vi "case_update_printer.vi"(0 "VISA resource name in":refnum<visa-resource-name>, 1 "Main VI reference":refnum<vi>, 5 "Refnum in":T2, 7 "message cluster":T1, 9 "initialized":bool, 11 "error in (no error)":errorcluster) -> (6 "Refnum out":T2, 8 "initialized out":bool, 15 "error out":errorcluster)   [LabVIEW 2020]
uses:
  <vilib>/Utility/config.llb/Config Data RefNum.ctl
  controls/message cluster.ctl
  64326d8d-66cc-4468-9ae1-7dc234c258b1.vi
  abe03f72-a603-4dcd-809d-10ef4235ec58.vi
  b926d721-a196-43c8-96cf-a21578f52920.vi
  db0f2e50-7a24-4501-afe9-f92d5168bb2c.vi
  168b0aa5-e037-40d0-9813-dbd61d4aeaf3.vi
  a9cd6c2e-b2c6-430f-85e8-9fbb4aaab0bd.vi
  13e36b39-ac3a-4ec8-9f6e-05db5e58b898.vi
  b8b0c841-a67c-40df-9bde-ad31628f9d82.vi
  <vilib>/Utility/config.llb/Read Key (String).vi
  <vilib>/Utility/config.llb/Read Key (Double).vi
  <vilib>/Utility/config.llb/NI_LVConfig.lvlib
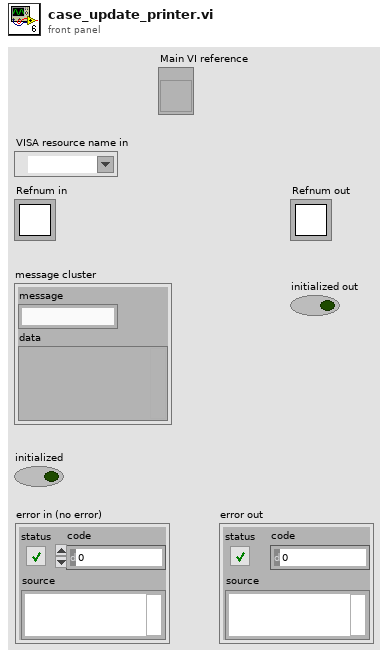
[diagram p1: front panel]
types:
  T1 = typedef "message cluster.ctl" = cluster{"message":string, "data":variant}
  T2 = typedef "NI_LVConfig.lvlib/Config Data RefNum.ctl" = refnum<k1>
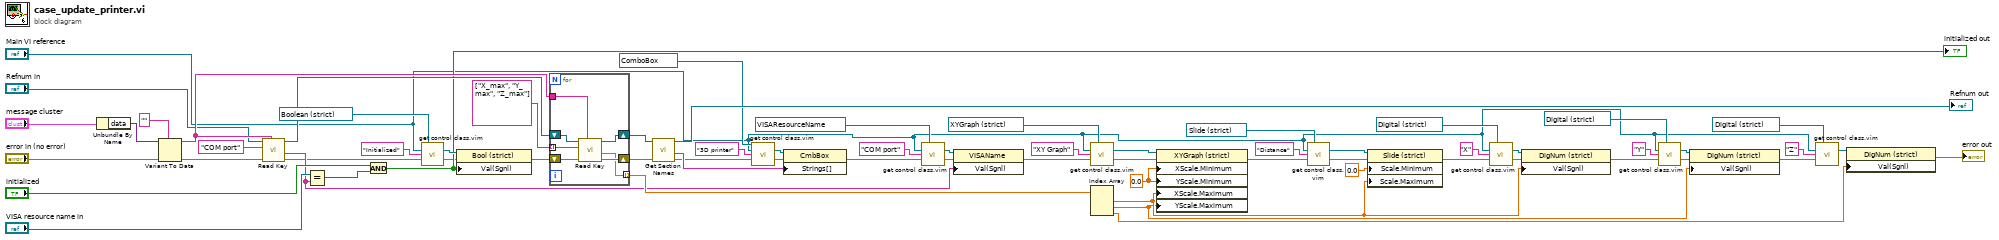
[diagram p0: block diagram]
diagram:
  w64 = 0.0 ("X Scale.Range:Minimum")
  n1 = Unbundle By Name("message cluster") -> ("data"=w47:variant)
  n2 = Variant To Data(error in="error in (no error)", type="", Variant=w47) -> (data=w57:string, error out=w50:errorcluster)
  n3 = call-poly <vilib>:"Read Key.vi"("section"=w57, "error in (no error)"=w50, "key"="COM port", "refnum"="Refnum in") -> ("error out"=w4:errorcluster, "value"=w15:string, "refnum out"=w56:T2)  [unwired: 4 in, 1 out]
  n4 = Equal?(x="VISA resource name in", y=w15) -> (x = y?=w63:bool)
  n5 = And(x="initialized", y=w63) -> (x .and. y?=w6:bool)
  "initialized out" <- w6
  n6 = call "get control class.vim"("Control class"=refnum<vi> refnum ("Initialized"), "Main VI reference"="Main VI reference", "Label"="Initialized", "error in (no error)"=w4) -> ("Control out"=w8:refnum<vi>, "error out"=w3:errorcluster)  [unwired: 10 in]
  n7 = property on="Property Node" class="Bool (strict)"(reference=w8, error in=w3, "Val(Sgnl)"=w6) -> (error out=w2:errorcluster)  [unwired: 1 out]
  n8 = for {
    tunnel: string[] ["X_max", "Y_max", "Z_max"] -> [w74] mode=indexing
    shift-right: [w71] -> w61
    shift-left: w2 -> [w72]
    shift-right: [w70] -> w59
    shift-left: w56 -> [w73]
    tunnel: [w69] -> w53 mode=indexing
    tunnel: w57 -> [w68]
    n9 = call-poly <vilib>:"Read Key.vi"("section"=w68, "error in (no error)"=w72, "key"=w74, "refnum"=w73) -> ("error out"=w71:errorcluster, "value"=w69:dbl, "refnum out"=w70:T2)  [unwired: 4 in, 1 out]
  }
  n10 = call <vilib>:"Get Section Names.vi"("error in (no error)"=w61, "refnum"=w59) -> ("error out"=w19:errorcluster, "section names"=w58:string[], "refnum out"=→"Refnum out":T2)  [unwired: 7 in]
  n11 = call "get control class.vim"("Control class"=refnum<vi> refnum ("3D printer"), "Main VI reference"="Main VI reference", "Label"="3D printer", "error in (no error)"=w19) -> ("Control out"=w36:refnum<vi>, "error out"=w18:errorcluster)  [unwired: 10 in]
  n12 = property on="Property Node" class="CmbBox"(reference=w36, error in=w18, "Strings[]"=w58) -> (error out=w20:errorcluster)  [unwired: 1 out]
  n13 = call "get control class.vim"("Control class"=refnum<vi> refnum ("Tab Control"), "Main VI reference"="Main VI reference", "Label"="COM port", "error in (no error)"=w20) -> ("Control out"=w44:refnum<vi>, "error out"=w43:errorcluster)  [unwired: 10 in]
  n14 = property on="Property Node" class="VISAName"(reference=w44, error in=w43, "Val(Sgnl)"=w15) -> (error out=w26:errorcluster)  [unwired: 1 out]
  n15 = call "get control class.vim"("Control class"=refnum<vi> refnum ("XY Graph"), "Main VI reference"="Main VI reference", "Label"="XY Graph", "error in (no error)"=w26) -> ("Control out"=w41:refnum<vi>, "error out"=w40:errorcluster)  [unwired: 10 in]
  n16 = Index Array(array=w53) -> (element #1=w66:dbl, element #2=w65:dbl, element #3=w54:dbl)  [unwired: 3 in]
  n17 = property on="Property Node" class="XYGraph (strict)"(reference=w41, error in=w40, "XScale.Minimum"=w64, "YScale.Minimum"=w64, "XScale.Maximum"=w66, "YScale.Maximum"=w65) -> (error out=w12:errorcluster)  [unwired: 1 out]
  n18 = call "get control class.vim"("Control class"=refnum<vi> refnum ("Distance"), "Main VI reference"="Main VI reference", "Label"="Distance", "error in (no error)"=w12) -> ("Control out"=w10:refnum<vi>, "error out"=w11:errorcluster)  [unwired: 10 in]
  n19 = property on="Property Node" class="Slide (strict)"(reference=w10, error in=w11, "Scale.Minimum"=0.0 ("Scale.Range:Minimum"), "Scale.Maximum"=w66) -> (error out=w25:errorcluster)  [unwired: 1 out]
  n20 = call "get control class.vim"("Control class"=refnum<vi> refnum ("X"), "Main VI reference"="Main VI reference", "Label"="X", "error in (no error)"=w25) -> ("Control out"=w33:refnum<vi>, "error out"=w24:errorcluster)  [unwired: 10 in]
  n21 = property on="Property Node" class="DigNum (strict)"(reference=w33, error in=w24, "Val(Sgnl)"=w66) -> (error out=w23:errorcluster)  [unwired: 1 out]
  n22 = call "get control class.vim"("Control class"=refnum<vi> refnum ("X"), "Main VI reference"="Main VI reference", "Label"="Y", "error in (no error)"=w23) -> ("Control out"=w30:refnum<vi>, "error out"=w22:errorcluster)  [unwired: 10 in]
  n23 = property on="Property Node" class="DigNum (strict)"(reference=w30, error in=w22, "Val(Sgnl)"=w65) -> (error out=w21:errorcluster)  [unwired: 1 out]
  n24 = call "get control class.vim"("Control class"=refnum<vi> refnum ("X"), "Main VI reference"="Main VI reference", "Label"="Z", "error in (no error)"=w21) -> ("Control out"=w27:refnum<vi>)  [unwired: 10 in, 1 out]
  n25 = property on="Property Node" class="DigNum (strict)"(reference=w27, "Val(Sgnl)"=w54) -> (error out=→"error out":errorcluster)  [unwired: 1 in, 1 out]
